vi "Tick Count (us) - Windows Only.vi"(11 "error in (no error)":errorcluster) -> (8 "micorsecond timer value":u64 format="%#.7f", 15 "error out":errorcluster)   [LabVIEW 2019]
doc: "Returns the current relative microsecond timer value from the high-resolution Windows counter.\n\nIf no high-resolution counter exists on the system, the function will return U64 MAX (18446744073709551615). Most modern architectures support a high-resolution counter."
uses:
  kernel32.dll
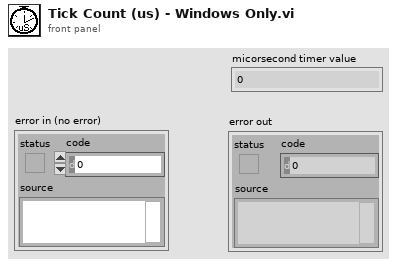
[diagram p1: front panel]
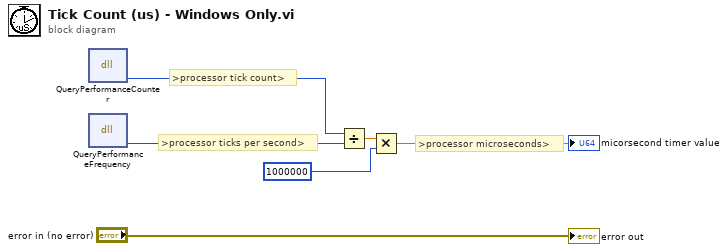
[diagram p0: block diagram]
diagram:
  # ">processor microseconds>"
  # ">processor ticks per second>"
  # ">processor tick count>"
  n1 = dll-call lib="kernel32.dll" fn="QueryPerformanceCounter"() -> ("pPerformanceCount"=w4:u64)  [unwired: 5 in, 2 out]
  n2 = dll-call lib="kernel32.dll" fn="QueryPerformanceFrequency"() -> ("pTicksPerSecond"=w3:u64)  [unwired: 5 in, 2 out]
  n3 = Divide(x=w4, y=w3) -> (x/y=w2:dbl)
  n4 = Multiply(x=w2, y=u64 1000000) -> (x*y=→"micorsecond timer value":dbl)
  "error out" <- "error in (no error)"
